vi "Write Single Cmd.vi"(8 "error in (no error)":errorcluster, 9 "Name":string, 10 "variant":variant, 11 "Modbus PLC in":refnum<class "Modbus PLC.lvclass">) -> (0 "error out":errorcluster, 3 "Modbus PLC out":refnum<class "Modbus PLC.lvclass">)   [LabVIEW 2023, in "Modbus PLC.lvlib" / "Modbus PLC.lvclass"]
uses:
  Modbus PLC.lvclass
  Modbus PLC.lvclass/Modbus PLC.ctl
  <vilib>/NI/Modbus Library/API/Master/Modbus Master.lvclass
  <vilib>/Utility/Data Type/NI_Data Type.lvlib
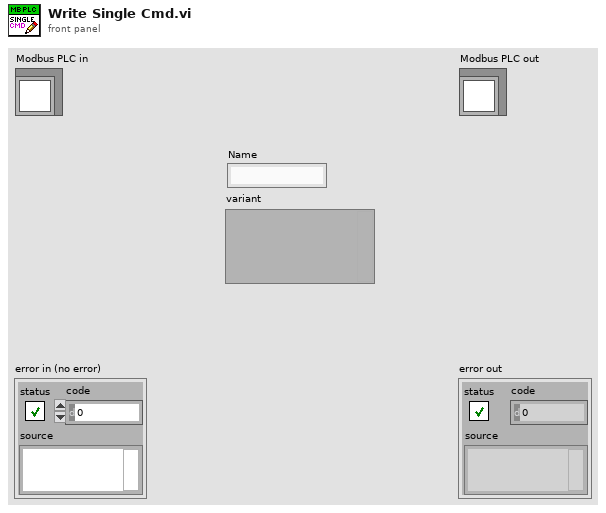
[diagram p1: front panel]
types:
  T1 = typedef "Modbus PLC.lvlib/Modbus PLC.lvclass/Input Map.ctl" = map{string, cluster{"Address":i32, "Data Type":enum16{"Int", "Float"}, "Reg Type":enum16{"Holding", "Input", "Coil"}}}
  T2 = cluster{"Address":i32, "Data Type":enum16{"Int", "Float"}, "Reg Type":enum16{"Holding", "Input", "Coil"}}
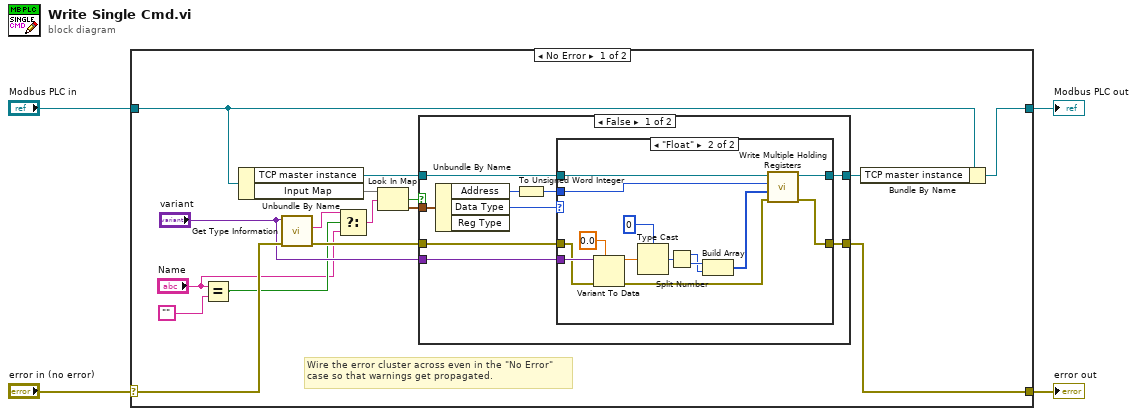
[diagram p0: block diagram]
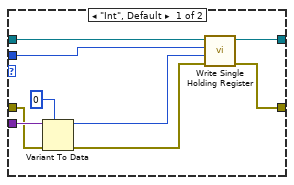
[diagram p2: hidden frame]
diagram:
  n1 = case shown="No Error" "error in (no error)" {
    selector: "error in (no error)" -> [w15 w56]
    tunnel: [w14 w56] -> w3
    tunnel: [w11 w55] -> w1
    tunnel: "Modbus PLC in" -> [w12 w55]
    frame No Error {
      # "Wire the error cluster across even in the \"No Error\"\ncase so that warnings get propagated."
      n2 = Equal?(x="Name", y="") -> (x = y?=w8:bool)
      n3 = Unbundle By Name(w12) -> ("TCP master instance"=w17:refnum<class "Modbus Master.lvclass">, "Input Map"=w20:T1)
      n4 = call <vilib>:"Get Type Information.vi"("error in (no error)"=w15, "variant"="variant") -> ("error out"=w16:errorcluster, "name"=w7:string)  [unwired: 5 in, 3 out]
      n5 = Select(t=w7, s=w8, f="Name") -> (s? t:f=w9:string)
      n6 = Look In Map(map=w20, key=w9) -> (key not found?=w18:bool, value=w19:T2)  [unwired: 1 in]
      n7 = case shown="False" w18 {
        tunnel: w19 -> [w29 _]
        tunnel: w17 -> [w27 w54]
        tunnel: "variant" -> [w26 _]
        tunnel: [w25 w54] -> w13
        tunnel: w16 -> [w22 w53]
        tunnel: [w21 w53] -> w14
        frame False {
          n8 = Unbundle By Name(w29) -> ("Address"=w24:i32, "Data Type"=w28:enum16{"Int", "Float"})  [unwired: 1 out]
          n9 = To Unsigned Word Integer(number=w24) -> (unsigned 16bit integer=w23:u16)
          n10 = case shown="\"Float\"" w28 {
            tunnel: w27 -> [w38 w52]
            tunnel: w26 -> [w37 w50]
            tunnel: [w34 w51] -> w25
            tunnel: w23 -> [w33 w46]
            tunnel: w22 -> [w31 w40]
            tunnel: [w32 w41] -> w21
            frame "Int", Default {
              n11 = Variant To Data(error in=w31, type=u16 0, Variant=w37) -> (data=w35:u16, error out=w30:errorcluster)
              n12 = call-dynamic "Write Single Holding Register.vi"("error in"=w30, "register to write"=w35, "address"=w33, "Modbus master in"=w38) -> ("error out"=w32:errorcluster, "Modbus master out"=w34:refnum<class "Modbus Master.lvclass">)  [unwired: 6 in]
            }
            frame "Float" {
              n13 = Variant To Data(error in=w40, type=sgl 0.0, Variant=w50) -> (data=w48:sgl, error out=w39:errorcluster)
              n14 = Type Cast(type=u32 0, x=w48) -> (*(type *) &x=w45:u32)
              n15 = Split Number(x=w45) -> (hi(x)=w43:u16, lo(x)=w44:u16)
              n16 = Build Array(w44, w43) -> (w42:u16[])
              n17 = call-dynamic "Write Multiple Holding Registers.vi"("error in"=w39, "registers to write"=w42, "starting address"=w46, "Modbus master in"=w52) -> ("error out"=w41:errorcluster, "Modbus master out"=w51:refnum<class "Modbus Master.lvclass">)  [unwired: 6 in]
            }
          }
        }
        frame True {
        }
      }
      n18 = Bundle By Name(cluster=w12, "TCP master instance"=w13) -> (w11:refnum<class "Modbus PLC.lvclass">)
    }
    frame Error {
    }
  }
  "error out" <- w3
  "Modbus PLC out" <- w1
